vi "Memory.Pointer.Write.Unsafe.1D.Bool.vi"(7 "count (-1: all)":i64=-1 format="%d elements", 8 "error in (no error)":errorcluster, 9 "offset (0)":u64 format="%d bytes", 10 "buffer in":bool[](array[boolean]), 11 "pointer in":refnum<class "Memory.Pointer.lvclass">) -> (0 "error out":errorcluster, 1 "offset out":u64 format="%d bytes", 2 "buffer out":bool[](array[boolean]), 3 "pointer out":refnum<class "Memory.Pointer.lvclass">)   [LabVIEW 2016, in "Memory Manager.lvlib" / "Memory.Pointer.lvclass"]
doc: "Writes <b>count</b> elements from the provided <b>buffer</b> to the address specified by <b>pointer + offset</b>.\n\n<b>Note:</b> This VI is <b>unsafe</b>.\n\nUnsafe means that it does not evaluate the size parameter of <b>pointer</b> to ensure that is inbounds of allocated memory before peforming a memory read/write. Reading/writing more data to a pointer than it has allocated can corrupt or crash LabVIEW. Only use this VI in scenarios where the <b>pointer</b> has been validated to be allocated to a correct size before calling this VI."
uses:
  Memory.Pointer.lvclass
  Memory.Pointer.lvclass/Memory.Pointer.ctl
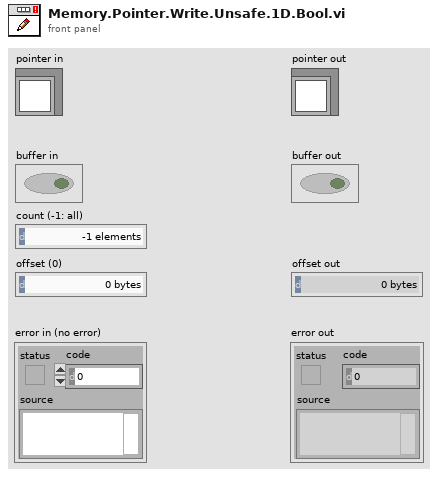
[diagram p1: front panel]
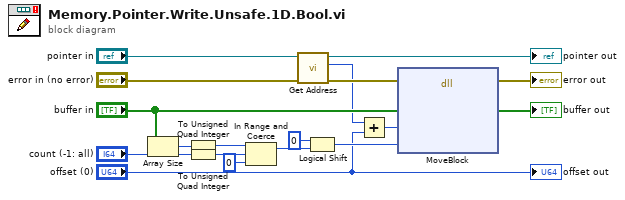
[diagram p0: block diagram]
diagram:
  n1 = Array Size(array="buffer in") -> (size(s)=w7:i32)
  n2 = To Unsigned Quad Integer(1:w7) -> (0:w2:u64)
  n3 = To Unsigned Quad Integer(1:"count (-1: all)") -> (0:w4:u64)
  n4 = In Range and Coerce(upper limit=w2, x=w4, lower limit=u64 0) -> (coerced(x)=w3:u64)  [unwired: 1 out]
  n5 = call "Get Address.vi"("error in (no error)"="error in (no error)", "Pointer in"="pointer in") -> ("error out"=w17:errorcluster, "address"=w1:u64, "Pointer out"=→"pointer out":refnum<class "Memory.Pointer.lvclass">)  [unwired: 7 in]
  n6 = Logical Shift(y=i16 0, x=w3) -> (x << y=w12:u64)
  n7 = Add(x=w1, y="offset (0)") -> (x+y=w10:u64)
  n8 = dll-call lib="LabVIEW" fn="MoveBlock"(error in=w17, "src"="buffer in", "dst"=w10, "size"=w12) -> (error out=→"error out":errorcluster, "src"=→"buffer out":bool[])  [unwired: 5 in, 1 out]
  "offset out" <- "offset (0)"
